vi "Parse WebSockets URL.vi"(8 "error in (no error)":errorcluster, 11 "WebSocket URL":string) -> (0 "error out":errorcluster, 1 "URI":string, 2 "host":string, 3 "protocol":string)   [LabVIEW 2013, in "WebSockets.lvlib" / "WebSocket Client.lvclass"]
uses:
  WebSocket Client.lvclass
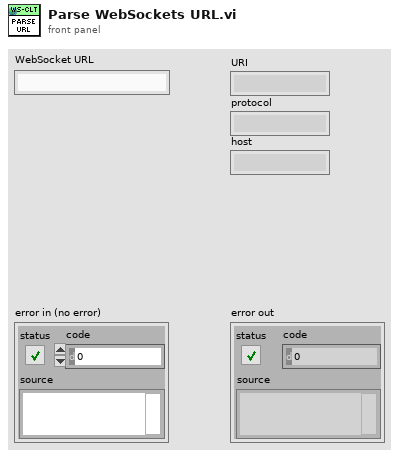
[diagram p1: front panel]
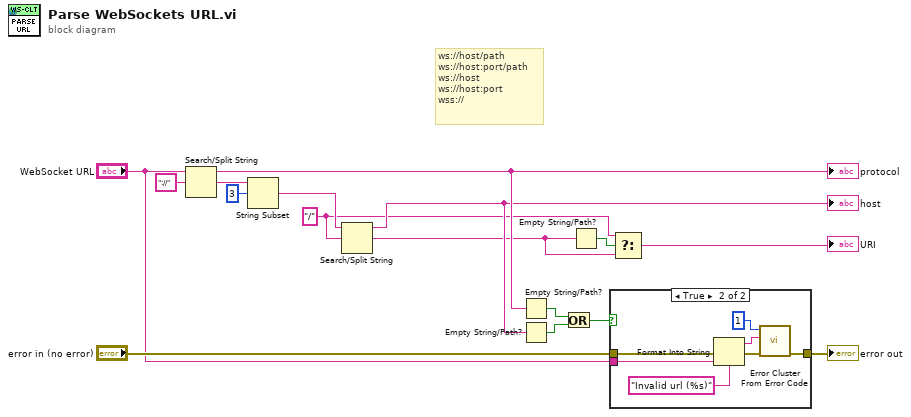
[diagram p0: block diagram]
diagram:
  w2 = "/" ("search string/char (-)")
  # "ws://host/path\nws://host:port/path\nws://host\nws://host:port\nwss://"
  n1 = Search/Split String(string="WebSocket URL", search string/char (-)="://") -> (substring before match=w11:string, match + rest of string=w13:string)  [unwired: 1 in, 1 out]
  "protocol" <- w11
  n2 = String Subset(string=w13, offset (0)=3) -> (substring=w12:string)  [unwired: 1 in]
  n3 = Search/Split String(string=w12, search string/char (-)=w2) -> (substring before match=w5:string, match + rest of string=w3:string)  [unwired: 1 in, 1 out]
  "host" <- w5
  n4 = Empty String/Path?(string/path=w11) -> (empty?=w10:bool)
  n5 = Empty String/Path?(string/path=w5) -> (empty?=w9:bool)
  n6 = Or(x=w10, y=w9) -> (x .or. y?=w6:bool)
  n7 = Empty String/Path?(string/path=w3) -> (empty?=w4:bool)
  n8 = case shown="True" w6 {
    tunnel: "error in (no error)" -> [w17 w24]
    tunnel: [w17 w23] -> w8
    tunnel: "WebSocket URL" -> [_ w20]
    frame False {
    }
    frame True {
      n9 = Format Into String(format string="Invalid url (%s)", error in=w24, w20) -> (resulting string=w21:string, error out=w22:errorcluster)  [unwired: 1 in]
      n10 = call <vilib>:"Error Cluster From Error Code.vi"("error in (no error)"=w22, "error message (\"\")"=w21, "error code (0)"=1) -> ("error out"=w23:errorcluster)  [unwired: 6 in]
    }
  }
  "error out" <- w8
  n11 = Select(t=w2, s=w4, f=w3) -> (s? t:f=→"URI":string)
